vi "HarvRoller.vi"(8 "HarvRollerBDesSpd":dbl, 9 "HarvRollerFDesSpd":dbl, 10 "HarvOutElev":dbl, 11 "HarvSetElev":i32) -> (1 "HarvOutRollerF 2":dbl, 2 "HarvOutRollerF":dbl, 3 "HarvShootEnable":bool)   [LabVIEW 2012]
panel:
  out "HarvOutElev":dbl
  in  "HarvSetElev":i32
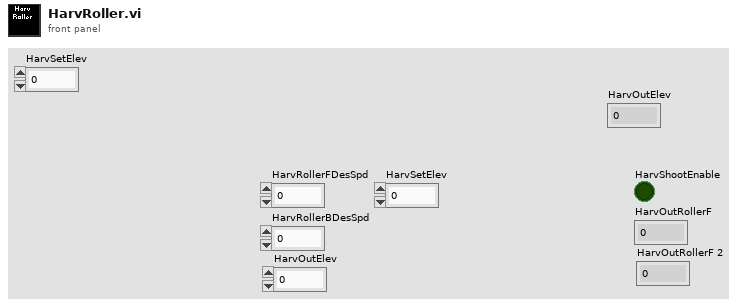
[diagram p1: front panel]
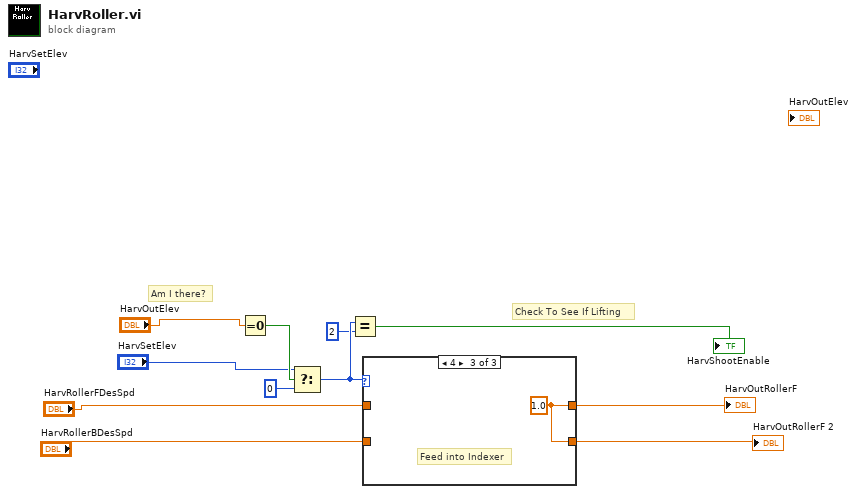
[diagram p0: block diagram]
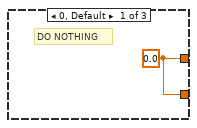
[diagram p2: hidden frame]
diagram:
  # "Am I there?"
  # "Check To See If Lifting"
  n1 = Equal To 0?(x="HarvOutElev") -> (x = 0?=w9:bool)
  n2 = Select(t="HarvSetElev", s=w9, f=0) -> (s? t:f=w7:i32)
  n3 = Equal?(x=w7, y=2) -> (x = y?=→"HarvShootEnable":bool)
  n4 = case shown="4" w7 {
    tunnel: [w12 w14 w15] -> w10
    tunnel: [w12 w13 w15] -> w5
    tunnel: "HarvRollerFDesSpd" -> [_ w14 _]
    tunnel: "HarvRollerBDesSpd" -> [_ w13 _]
    frame 0, Default {
      w12 = 0.0 ("HarvRollerFDesSpd")
      # "DO NOTHING"
    }
    frame 1..3 {
    }
    frame 4 {
      w15 = 1.0 ("HarvRollerFDesSpd")
      # "Feed into Indexer"
    }
  }
  "HarvOutRollerF" <- w10
  "HarvOutRollerF 2" <- w5
